vi "write_file.vi"(6 "Data File":path, 7 "error in (no error)":errorcluster {"code" format="%.0x"}, 8 "Y Axis Data":dbl[](array[numeric]), 9 "Step Size":dbl, 10 "Initial Value":dbl) -> (0 "error out":errorcluster {"code" format="%.0x"}, 2 "xArray":dbl[](array[numeric]))   [LabVIEW 2015]
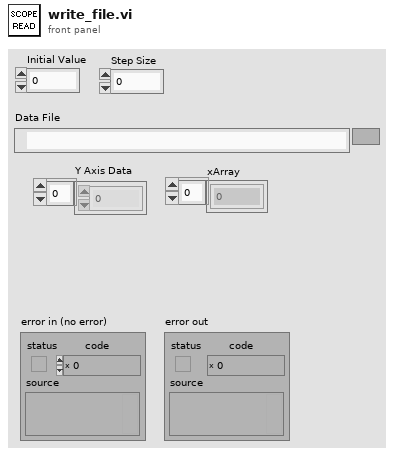
[diagram p1: front panel]
types:
  T1 = enum16{"open", "replace", "create", "open or create", "replace or create", "replace or create with confirmation"}
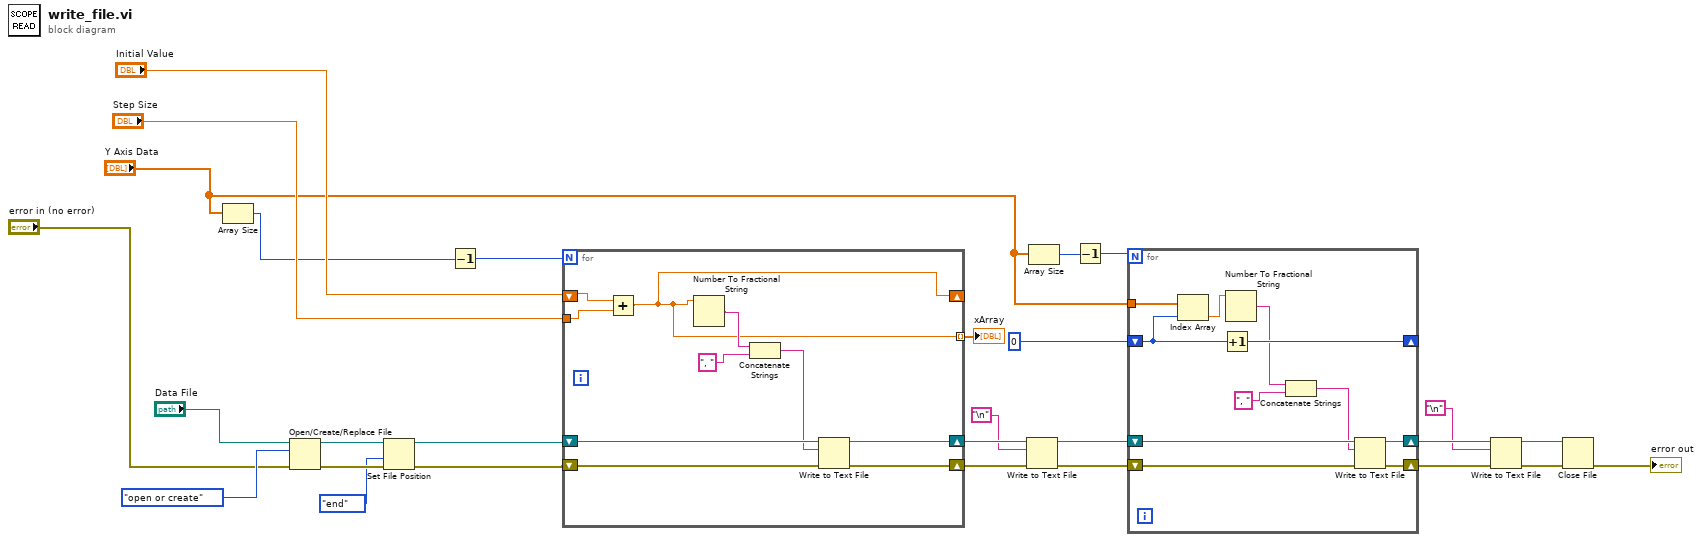
[diagram p0: block diagram]
diagram:
  n1 = Array Size(array="Y Axis Data") -> (size(s)=w3:i32)
  n2 = Open/Create/Replace File(file path (use dialog)="Data File", error in="error in (no error)", operation (0:open)=T1."open or create") -> (refnum out=w28:refnum<file>, error out=w27:errorcluster)  [unwired: 3 in, 1 out]
  n3 = Set File Position(refnum=w28, from (0:start)=enum16{"start", "end", "current"}."end", error in=w27) -> (refnum out=w8:refnum<file>, error out=w7:errorcluster)  [unwired: 1 in]
  n4 = Decrement(x=w3) -> (x-1=w23:i32)
  n5 = for {
    N: w23 -> [_]
    tunnel: "Step Size" -> [w38]
    shift-right: [w29] -> _
    shift-left: "Initial Value" -> [w37]
    shift-right: [w32] -> w19
    shift-left: w8 -> [w36]
    shift-right: [w31] -> w18
    shift-left: w7 -> [w35]
    tunnel: [w29] -> w1 mode=indexing
    n6 = Add(x=w37, y=w38) -> (x+y=w29:dbl)
    n7 = Number To Fractional String(number=w29) -> (F-format string=w30:string)  [unwired: 3 in]
    n8 = Concatenate Strings(w30, ", ") -> (w33:string)
    n9 = Write to Text File(file (use dialog)=w36, text=w33, error in=w35) -> (refnum out=w32:refnum<file>, error out=w31:errorcluster)  [unwired: 1 in, 1 out]
  }
  "xArray" <- w1
  n10 = Write to Text File(file (use dialog)=w19, text="\n", error in=w18) -> (refnum out=w13:refnum<file>, error out=w12:errorcluster)  [unwired: 1 in, 1 out]
  n11 = Array Size(array="Y Axis Data") -> (size(s)=w15:i32)
  n12 = Decrement(x=w15) -> (x-1=w16:i32)
  n13 = for {
    N: w16 -> [_]
    tunnel: "Y Axis Data" -> [w49]
    shift-right: [w47] -> _
    shift-left: 0 -> [w48]
    shift-right: [w42] -> w11
    shift-left: w13 -> [w45]
    shift-right: [w41] -> w10
    shift-left: w12 -> [w44]
    n14 = Index Array(array=w49, index=w48) -> (element=w39:dbl)
    n15 = Increment(x=w48) -> (x+1=w47:i32)
    n16 = Number To Fractional String(number=w39) -> (F-format string=w40:string)  [unwired: 3 in]
    n17 = Concatenate Strings(w40, ", ") -> (w43:string)
    n18 = Write to Text File(file (use dialog)=w45, text=w43, error in=w44) -> (refnum out=w42:refnum<file>, error out=w41:errorcluster)  [unwired: 1 in, 1 out]
  }
  n19 = Write to Text File(file (use dialog)=w11, text="\n", error in=w10) -> (refnum out=w20:refnum<file>, error out=w22:errorcluster)  [unwired: 1 in, 1 out]
  n20 = Close File(refnum=w20, error in=w22) -> (error out=→"error out":errorcluster)  [unwired: 1 out]
